vi "ma-resample unevenly sampled input (linear interpolation).vi"(0 "X-array in":dbl[](array[numeric]) format="%.2p", 5 "Y-array in":dbl[](array[numeric]) format="%.2p", 7 "dt":dbl=1.0 format="%.2p", 9 "t0":dbl format="%.2p", 11 "error in":errorcluster) -> (4 "X-array out":dbl[](array[numeric]) format="%.2p", 6 "Y-array out":dbl[](array[numeric]) format="%.2p", 8 "evenly sampled waveform out":waveform(dbl), 10 "used t0":dbl format="%.2p", 14 "t0 adjusted warning":bool, 15 "error out":errorcluster)   [LabVIEW 2020, in "NI_MAPro.lvlib"]
doc: "This VI re-samples an unevenly sampled input signal to an evenly sampled waveform according to specified t0 and dt. If the specified t0 value is less than the first value of input X-array (that is the timestamp of the first input sample), then the VI will coerce t0 to the first valid value (greater than X(0)) that also fulfill the relation:\n\nT0_adjusted - t0_in = n * dt_in\n\nThis guarranty that any later comparison of waveforms will be correct with repsect to absolute time."
uses:
  NI_MAPro.lvlib
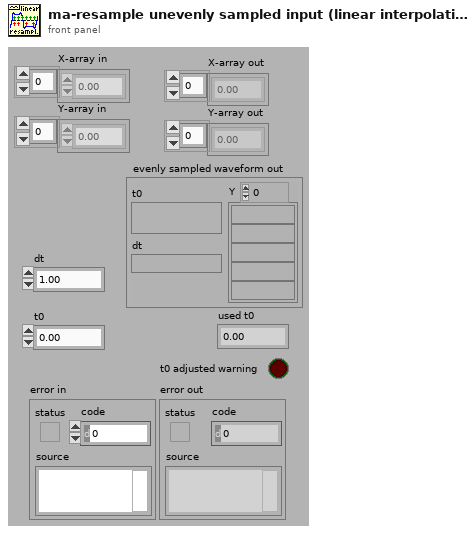
[diagram p1: front panel]
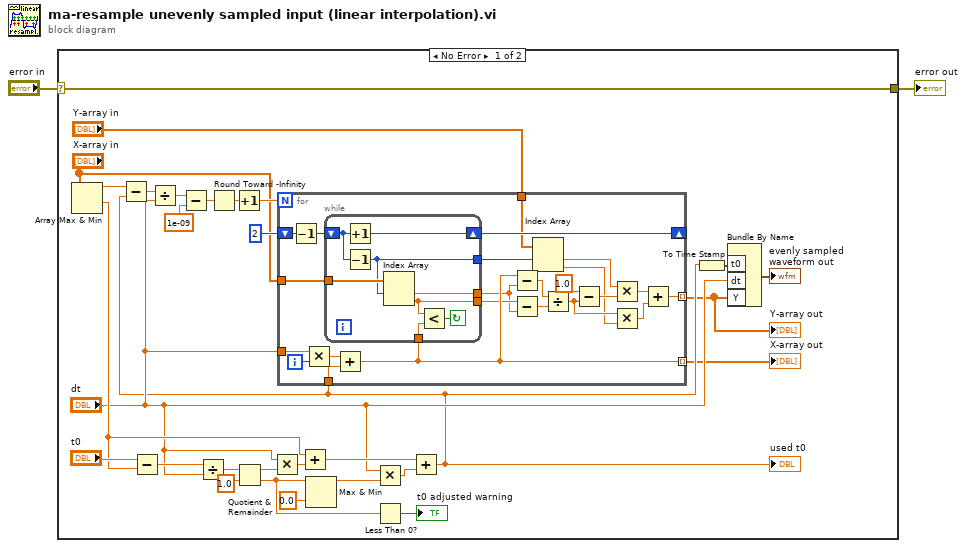
[diagram p0: block diagram]
diagram:
  n1 = case shown="No Error" "error in" {
    selector: "error in" -> [w4 w64]
    tunnel: [w4 w64] -> w1
    frame No Error {
      n2 = Array Max & Min(array="X-array in") -> (max value=w17:dbl, min value=w14:dbl)  [unwired: 2 out]
      n3 = Subtract(x="t0", y=w14) -> (x-y=w29:dbl)
      n4 = Divide(x=w29, y="dt") -> (x/y=w31:dbl)
      n5 = Quotient & Remainder(x=w31, y=1.0) -> (x-y*floor(x/y)=w20:dbl, floor(x/y)=w22:dbl)
      n6 = Multiply(x="dt", y=w20) -> (x*y=w28:dbl)
      n7 = Add(x=w14, y=w28) -> (x+y=w25:dbl)
      n8 = Max & Min(x=w22, y=0.0) -> (max(x,y)=w24:dbl)  [unwired: 1 out]
      n9 = Multiply(x="dt", y=w24) -> (x*y=w27:dbl)
      n10 = Less Than 0?(x=w22) -> (x < 0?=→"t0 adjusted warning":bool)
      n11 = Add(x=w25, y=w27) -> (x+y=w12:dbl)
      "used t0" <- w12
      n12 = Subtract(x=w17, y=w12) -> (x-y=w18:dbl)
      n13 = Divide(x=w18, y="dt") -> (x/y=w11:dbl)
      n14 = Subtract(x=w11, y=1e-09) -> (x-y=w9:dbl)
      n15 = Round Toward -Infinity(1:w9) -> (0:w16:dbl)
      n16 = Increment(x=w16) -> (x+1=w15:dbl)
      n17 = for {
        N: w15 -> [_]
        tunnel: "dt" -> [w54]
        tunnel: w12 -> [w52]
        tunnel: "X-array in" -> [w51]
        shift-right: [w49] -> _
        shift-left: 2 -> [w50]
        tunnel: [w45] -> w7 mode=indexing
        tunnel: "Y-array in" -> [w47]
        tunnel: [w33] -> w8 mode=indexing
        i -> [w55]
        n18 = Decrement(x=w50) -> (x-1=w48:i32)
        n19 = Multiply(x=w54, y=w55) -> (x*y=w53:dbl)
        n20 = Add(x=w53, y=w52) -> (x+y=w45:dbl)
        n21 = while {
          tunnel: w51 -> [w63]
          shift-right: [w61] -> w49
          shift-left: w48 -> [w58]
          tunnel: w45 -> [w62]
          tunnel: [w57] -> w46
          tunnel: [w59] -> w42
          tunnel: [w60] -> w43
          stop <- w56 continue-if-true
          n22 = Increment(x=w58) -> (x+1=w61:i32)
          n23 = Decrement(x=w58) -> (x-1=w57:i32)
          n24 = Index Array(array=w63, index #1=w57) -> (element #1=w59:dbl, element #2=w60:dbl)  [unwired: 1 in]
          n25 = Less?(x=w60, y=w62) -> (x < y?=w56:bool)
        }
        n26 = Subtract(x=w45, y=w42) -> (x-y=w44:dbl)
        n27 = Subtract(x=w43, y=w42) -> (x-y=w41:dbl)
        n28 = Index Array(array=w47, index #1=w46) -> (element #1=w39:dbl, element #2=w36:dbl)  [unwired: 1 in]
        n29 = Divide(x=w44, y=w41) -> (x/y=w37:dbl)
        n30 = Subtract(x=1.0, y=w37) -> (x-y=w38:dbl)
        n31 = Multiply(x=w39, y=w38) -> (x*y=w35:dbl)
        n32 = Multiply(x=w37, y=w36) -> (x*y=w34:dbl)
        n33 = Add(x=w35, y=w34) -> (x+y=w33:dbl)
      }
      "X-array out" <- w7
      "Y-array out" <- w8
      n34 = To Time Stamp(1:w12) -> (0:w3:timestamp)
      n35 = Bundle By Name("t0"=w3, "dt"="dt", "Y"=w8) -> (→"evenly sampled waveform out":waveform(dbl))  [unwired: 1 in]
    }
    frame Error {
    }
  }
  "error out" <- w1
